vi "Distance from XY Delta.vi"(11 "Delta Point":cluster{dbl, dbl}) -> (3 "Distance":dbl)   [LabVIEW 2019]
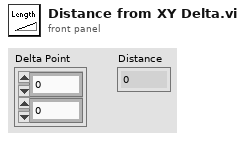
[diagram p1: front panel]
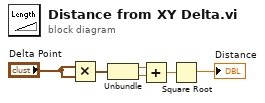
[diagram p0: block diagram]
diagram:
  n1 = Multiply(x="Delta Point", y="Delta Point") -> (x*y=w1:cluster{dbl, dbl})
  n2 = Unbundle(w1) -> (w2:dbl, w3:dbl)
  n3 = Add(x=w2, y=w3) -> (x+y=w4:dbl)
  n4 = Square Root(x=w4) -> (sqrt(x)=→"Distance":dbl)
